vi "供电开关.vi"(8 "error in (no error)":errorcluster, 10 "OUT1供电开关":bool) -> (0 "error out":errorcluster)   [LabVIEW 2016, in "斯坦道多参数.lvlib"]
uses:
  <vilib>/Instr/_visa.llb/VISA Configure Serial Port (Instr).vi
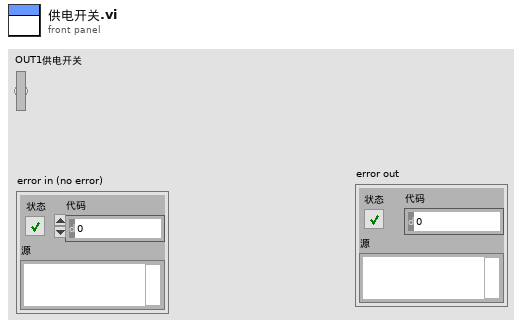
[diagram p1: front panel]
types:
  T1 = cluster{"VISA resource name":refnum<visa-resource-name>, "启用":bool, "开/关":bool}
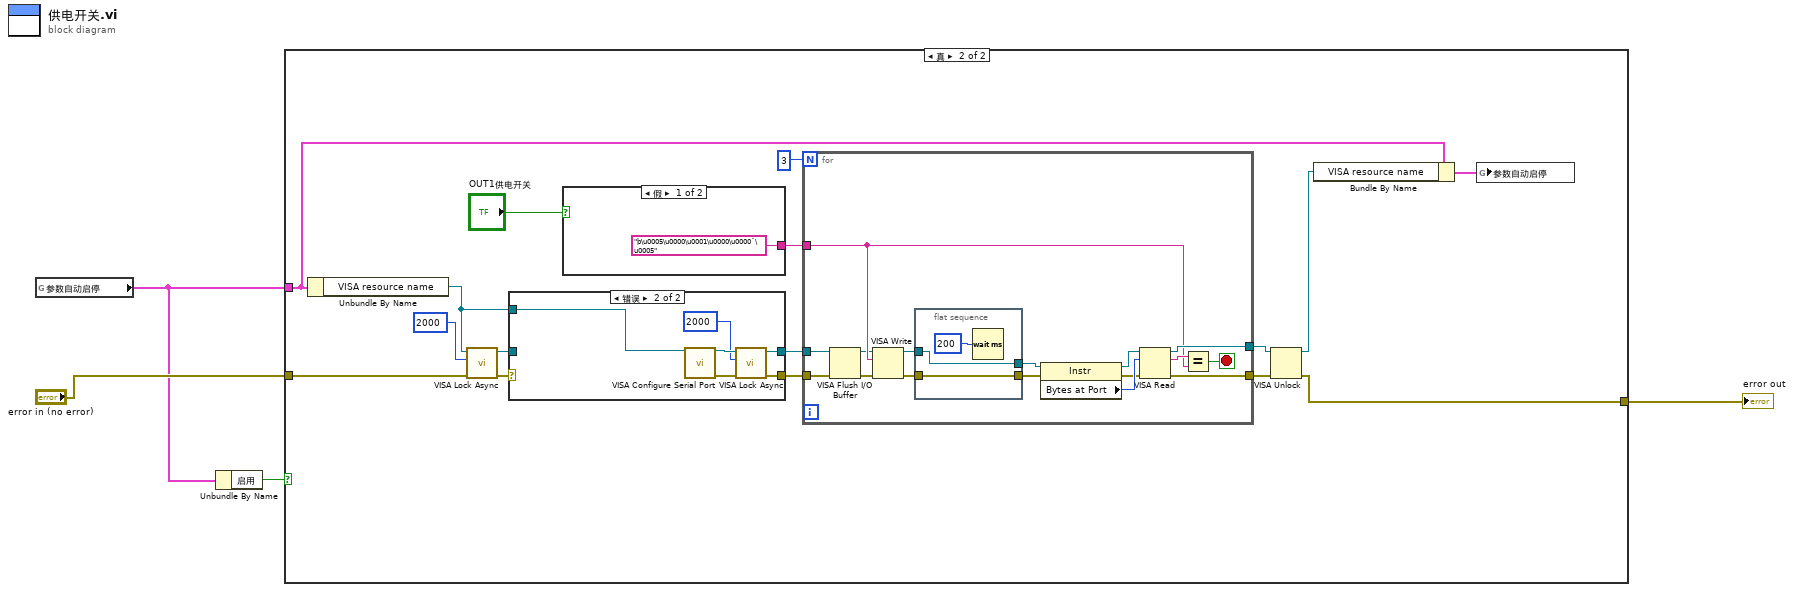
[diagram p0: block diagram]
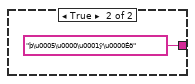
[diagram p4: hidden frame]
diagram:
  n1 = global read "断电保存变量.vi" "参数自动启停"() -> (w1:T1)
  n2 = Unbundle By Name(w1) -> ("启用"=w4:bool)
  n3 = case shown="真" w4 {
    tunnel: w1 -> [_ w9]
    tunnel: [w5 w8] -> w3
    tunnel: "error in (no error)" -> [w5 w7]
    frame False {
    }
    frame True {
      n4 = Unbundle By Name(w9) -> ("VISA resource name"=w10:refnum<visa-resource-name>)
      n5 = call <vilib>:"VISA Lock Async.vi"("error in (no error)"=w7, "timeout (0)"=u32 2000, "VISA resource name"=w10) -> ("error out"=w16:errorcluster, "VISA resource name out"=w15:refnum<visa-resource-name>)  [unwired: 6 in, 1 out]
      n6 = case shown="错误" w16 {
        selector: w16 -> [w22 _]
        tunnel: [w23 w27] -> w14
        tunnel: w15 -> [w23 _]
        tunnel: [w22 w26] -> w13
        tunnel: w10 -> [_ w24]
        frame No Error {
        }
        frame Error {
          n7 = call-poly "VISA Configure Serial Port"("VISA resource name"=w24) -> ("VISA resource name out"=w28:refnum<visa-resource-name>, "error out"=w29:errorcluster)  [unwired: 13 in]
          n8 = call <vilib>:"VISA Lock Async.vi"("error in (no error)"=w29, "timeout (0)"=u32 2000, "VISA resource name"=w28) -> ("error out"=w26:errorcluster, "VISA resource name out"=w27:refnum<visa-resource-name>)  [unwired: 6 in, 1 out]
        }
      }
      n9 = case shown="假" "OUT1供电开关" {
        tunnel: ["þ\u0005\u0000\u0001\u0000\u0000ˆ\u0005" ("write buffer") "þ\u0005\u0000\u0001ÿ\u0000Éõ" ("write buffer")] -> w20
        frame False {
        }
        frame True {
        }
      }
      n10 = for {
        N: 3 -> [_]
        tunnel: w20 -> [w32]
        tunnel: [w37] -> w17
        tunnel: w14 -> [w36]
        tunnel: w13 -> [w35]
        tunnel: [w38] -> w18
        stop <- w31 stop-if-true
        n11 = VISA Flush I/O Buffer(VISA resource name=w36, error in (no error)=w35) -> (VISA resource name out=w30:refnum<visa-resource-name>, error out=w34:errorcluster)  [unwired: 1 in]
        n12 = VISA Write(VISA resource name=w30, write buffer=w32, error in (no error)=w34) -> (VISA resource name out=w45:refnum<visa-resource-name>, error out=w44:errorcluster)  [unwired: 1 out]
        n13 = flat-sequence {
          tunnel: w45 -> [w48]
          tunnel: w44 -> [w46]
          tunnel: [w48] -> w43
          tunnel: [w46] -> w42
          frame #0 {
            n14 = Wait (ms)(milliseconds to wait=u32 200) -> ()  [unwired: 1 out]
          }
        }
        n15 = property class="Instr"(reference=w43, error in=w42) -> (reference out=w41:refnum<visa-resource-name>, error out=w39:errorcluster, "Bytes at Port"=w40:u32)
        n16 = VISA Read(VISA resource name=w41, byte count=w40, error in (no error)=w39) -> (VISA resource name out=w37:refnum<visa-resource-name>, read buffer=w33:string, error out=w38:errorcluster)  [unwired: 1 out]
        n17 = Equal?(x=w33, y=w32) -> (x = y?=w31:bool)
      }
      n18 = VISA Unlock(8:w18, 11:w17) -> (0:w8:errorcluster, 3:w11:refnum<visa-resource-name>)
      n19 = Bundle By Name(cluster=w9, "VISA resource name"=w11) -> (w6:T1)
      n20 = global write "断电保存变量.vi" "参数自动启停"(w6) -> ()
    }
  }
  "error out" <- w3
